vi "Modify Joystick Values.vi"(2 "Joystick Input 2":dbl, 3 "Quadrify the values":bool, 4 "Joystick Input 1":dbl) -> (0 "Joystick Output 2":dbl, 1 "Joystick Output 1":dbl)   [LabVIEW 2015]
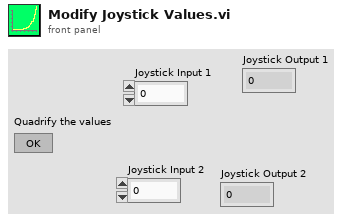
[diagram p1: front panel]
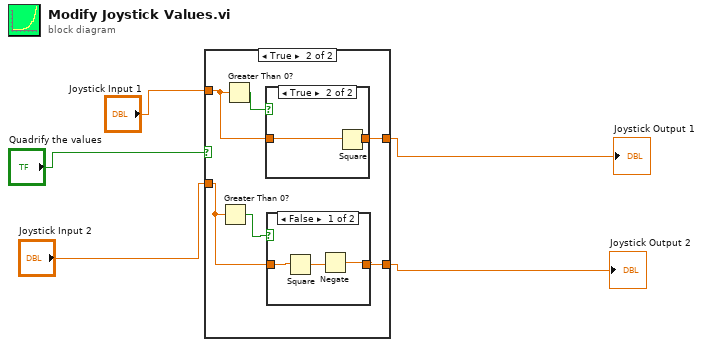
[diagram p0: block diagram]
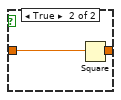
[diagram p3: hidden frame]
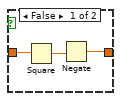
[diagram p4: hidden frame]
diagram:
  n1 = case shown="True" "Quadrify the values" {
    tunnel: "Joystick Input 1" -> [w7 w12]
    tunnel: "Joystick Input 2" -> [w6 w10]
    tunnel: [w7 w9] -> w3
    tunnel: [w6 w8] -> w2
    frame False {
    }
    frame True {
      n2 = Greater Than 0?(x=w10) -> (x > 0?=w11:bool)
      n3 = Greater Than 0?(x=w12) -> (x > 0?=w13:bool)
      n4 = case shown="True" w13 {
        tunnel: w12 -> [w21 w23]
        tunnel: [w19 w22] -> w9
        frame False {
          n5 = Square(x=w21) -> (x^2=w20:dbl)
          n6 = Negate(x=w20) -> (-x=w19:dbl)
        }
        frame True {
          n7 = Square(x=w23) -> (x^2=w22:dbl)
        }
      }
      n8 = case shown="False" w11 {
        tunnel: w10 -> [w16 w18]
        tunnel: [w14 w17] -> w8
        frame False {
          n9 = Square(x=w16) -> (x^2=w15:dbl)
          n10 = Negate(x=w15) -> (-x=w14:dbl)
        }
        frame True {
          n11 = Square(x=w18) -> (x^2=w17:dbl)
        }
      }
    }
  }
  "Joystick Output 1" <- w3
  "Joystick Output 2" <- w2
